vi "Get LV Version Year.vi"(8 "error in (no error)":errorcluster) -> (0 "error out":errorcluster, 3 "Year":string)   [LabVIEW 2011, in "Sensor Simulation Custom Device.lvlib"]
uses:
  Sensor Simulation Custom Device.lvlib
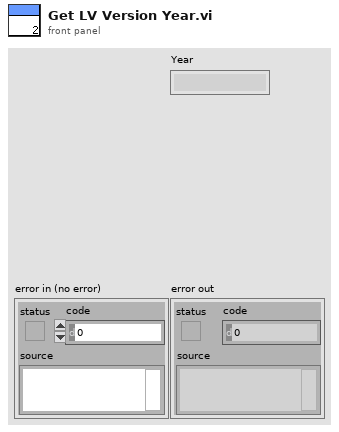
[diagram p1: front panel]
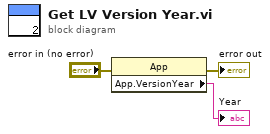
[diagram p0: block diagram]
diagram:
  n1 = property class="App"(error in="error in (no error)") -> (error out=→"error out":errorcluster, "App.VersionYear"=→"Year":string)  [unwired: 1 in, 1 out]
